vi "Register File.vi"(8 "Error In":errorcluster, 10 "Sequence File In":refnum<k7>, 11 "Application Manager In":refnum<k7>) -> (0 "Error out":errorcluster, 1 "Events":refnum<k27>[](array[refnum]), 2 "Sequence File Out":refnum<k7>, 3 "Application Manager Out":refnum<k7>)   [LabVIEW 2021, in "Seq Edit Quick Drop.lvlib"]
uses:
  Seq Edit Quick Drop.lvlib
  Connection Type.ctl
  Event Data.ctl
  Event Handler - Sequence View - Key Down.vi
  Event Handler - Sequence List - Key Up.vi
  Event Handler - Variables View - Key Down.vi
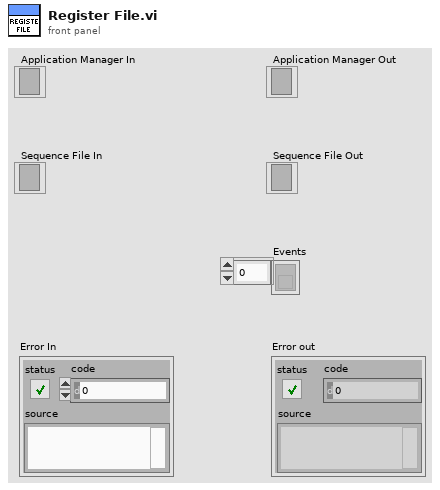
[diagram p1: front panel]
types:
  T1 = typedef "Seq Edit Quick Drop.lvlib/Event Data.ctl" = cluster{"Engine ID":string, "ID":i32}
  T2 = typedef "Seq Edit Quick Drop.lvlib/Connection Type.ctl" = enum16{"SequenceView", "SequenceList", "VariablesView"}
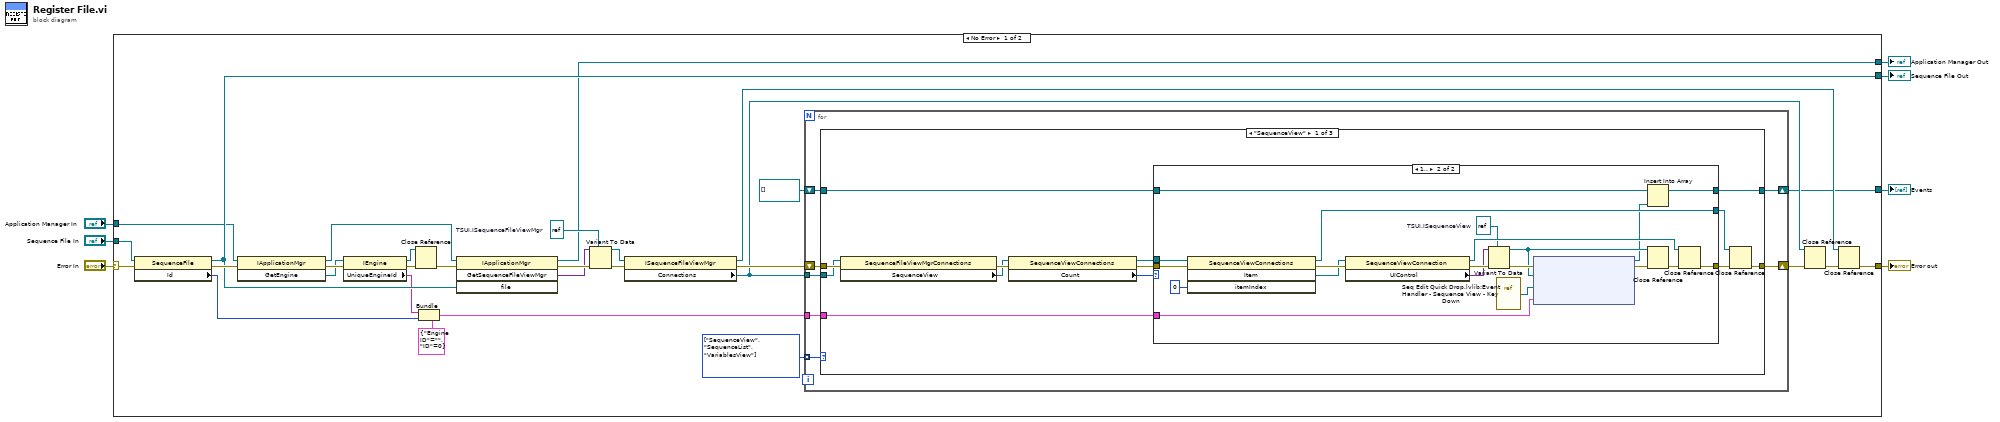
[diagram p0: block diagram]
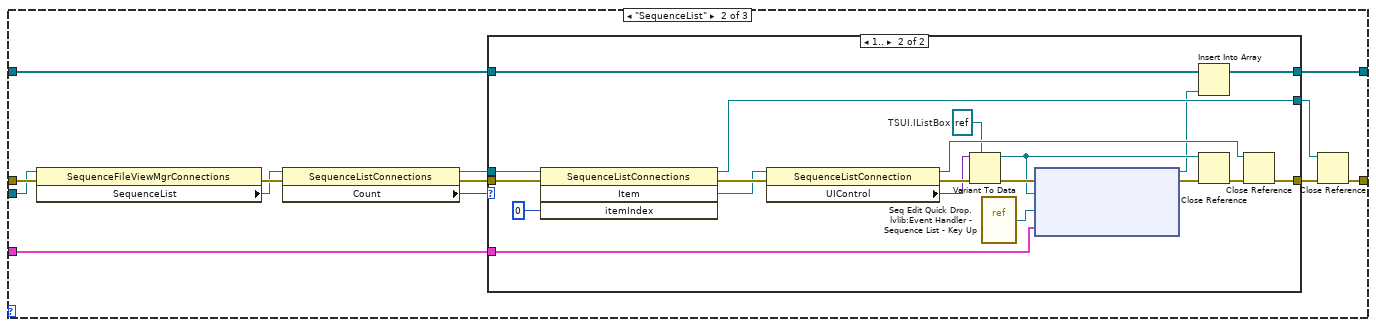
[diagram p3: hidden frame]
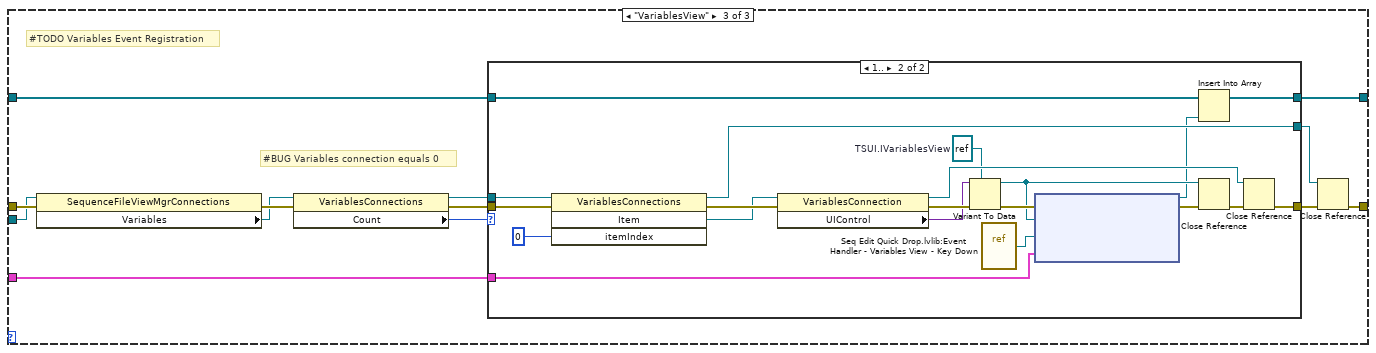
[diagram p5: hidden frame]
diagram:
  n1 = case shown="No Error" "Error In" {
    selector: "Error In" -> [w28 w155]
    tunnel: [w29 w155] -> w4
    tunnel: [w26 w154] -> w2
    tunnel: [w18 _] -> w3
    tunnel: "Application Manager In" -> [w17 w154]
    tunnel: "Sequence File In" -> [w20 w153]
    tunnel: [w35 w153] -> w1
    frame No Error {
      w25 = T2[] [enum."SequenceView", enum."SequenceList", enum."VariablesView"] items=["SequenceView", "SequenceList", "VariablesView"]
      w32 = refnum<k7> refnum  # TSUI.ISequenceFileViewMgr
      n2 = property class="SequenceFile"(reference=w20, error in=w28) -> (reference out=w35:refnum<k7>, error out=w36:errorcluster, "Id"=w10:i32)
      n3 = invoke class="IApplicationMgr" method="GetEngine"(reference=w17, error in=w36) -> (reference out=w15:refnum<k7>, error out=w37:errorcluster, "GetEngine"=w16:refnum<k7>)  [unwired: 1 in]
      n4 = property class="IEngine"(reference=w16, error in=w37) -> (reference out=w12:refnum<k7>, error out=w14:errorcluster, "UniqueEngineId"=w9:string)
      n5 = Close Reference(reference=w12, error in (no error)=w14) -> (error out=w13:errorcluster)
      n6 = Bundle(cluster=T1 {"Engine ID"="", "ID"=0}, "Engine ID"=w9, "ID"=w10) -> (w8:T1)
      n7 = invoke class="IApplicationMgr" method="GetSequenceFileViewMgr"(reference=w15, error in=w13, "file"=w35) -> (reference out=w26:refnum<k7>, error out=w34:errorcluster, "GetSequenceFileViewMgr"=w33:variant)  [unwired: 1 in, 1 out]
      n8 = Variant To Data(error in=w34, type=w32, Variant=w33) -> (data=w30:refnum<k7>, error out=w31:errorcluster)
      n9 = property class="ISequenceFileViewMgr"(reference=w30, error in=w31) -> (reference out=w27:refnum<k7>, error out=w24:errorcluster, "Connections"=w21:refnum<k7>)
      n10 = for {
        tunnel: w25 -> [w44] mode=indexing
        shift-right: [w41] -> w23
        shift-left: w24 -> [w42]
        tunnel: w21 -> [w43]
        shift-right: [w39] -> w18
        shift-left: refnum<k27>[] [] -> [w40]
        tunnel: w8 -> [w38]
        n11 = case shown="\"SequenceView\"" w44 {
          tunnel: w43 -> [w56 w92 w128]
          tunnel: w42 -> [w57 w93 w129]
          tunnel: [w47 w84 w120] -> w41
          tunnel: [w48 w82 w118] -> w39
          tunnel: w40 -> [w46 w83 w119]
          tunnel: w38 -> [w45 w81 w117]
          frame "SequenceView" {
            n12 = property class="SequenceFileViewMgrConnections"(reference=w56, error in=w57) -> (error out=w55:errorcluster, "SequenceView"=w54:refnum<k7>)  [unwired: 1 out]
            n13 = property class="SequenceViewConnections"(reference=w54, error in=w55) -> (reference out=w51:refnum<k7>, error out=w52:errorcluster, "Count"=w53:i32)
            n14 = case shown="1.." w53 {
              tunnel: w52 -> [w60 w77]
              tunnel: w51 -> [w59 w76]
              tunnel: [w60 w67] -> w50
              tunnel: [w59 w69] -> w49
              tunnel: [w58 w64] -> w48
              tunnel: w46 -> [w58 w65]
              tunnel: w45 -> [_ w61]
              frame Default {
              }
              frame 1.. {
                w73 = refnum<k7> refnum  # TSUI.ISequenceView
                n15 = invoke class="SequenceViewConnections" method="Item"(reference=w76, error in=w77, "itemIndex"=0) -> (reference out=w69:refnum<k7>, error out=w72:errorcluster, "Item"=w71:refnum<k7>)  [unwired: 1 in, 1 out]
                n16 = property class="SequenceViewConnection"(reference=w71, error in=w72) -> (reference out=w80:refnum<k7>, error out=w78:errorcluster, "UIControl"=w74:variant)
                n17 = Variant To Data(error in=w78, type=w73, Variant=w74) -> (data=w66:refnum<k7>, error out=w79:errorcluster)
                n18 = vi-ref "Seq Edit Quick Drop.lvlib:Event Handler - Sequence View - Key Down.vi"() -> ("vi reference"=w62:refnum<vi>)
                n19 = node(w79, w66, w62, w61) -> (w63:refnum<k27>, w70:errorcluster)  [unwired: 1 in]
                n20 = Insert Into Array(array=w65, new element=w63) -> (w64:refnum<k27>[])  [unwired: 1 in]
                n21 = Close Reference(reference=w66, error in (no error)=w70) -> (error out=w68:errorcluster)
                n22 = Close Reference(reference=w80, error in (no error)=w68) -> (error out=w67:errorcluster)
              }
            }
            n23 = Close Reference(reference=w49, error in (no error)=w50) -> (error out=w47:errorcluster)
          }
          frame "SequenceList" {
            n24 = property class="SequenceFileViewMgrConnections"(reference=w92, error in=w93) -> (error out=w91:errorcluster, "SequenceList"=w90:refnum<k7>)  [unwired: 1 out]
            n25 = property class="SequenceListConnections"(reference=w90, error in=w91) -> (reference out=w87:refnum<k7>, error out=w88:errorcluster, "Count"=w89:i32)
            n26 = case shown="1.." w89 {
              tunnel: w88 -> [w96 w113]
              tunnel: w87 -> [w95 w112]
              tunnel: [w96 w103] -> w86
              tunnel: [w95 w105] -> w85
              tunnel: w83 -> [w94 w101]
              tunnel: [w94 w99] -> w82
              tunnel: w81 -> [_ w98]
              frame Default {
              }
              frame 1.. {
                w109 = refnum<k7> refnum  # TSUI.IListBox
                n27 = invoke class="SequenceListConnections" method="Item"(reference=w112, error in=w113, "itemIndex"=0) -> (reference out=w105:refnum<k7>, error out=w108:errorcluster, "Item"=w107:refnum<k7>)  [unwired: 1 in, 1 out]
                n28 = property class="SequenceListConnection"(reference=w107, error in=w108) -> (reference out=w116:refnum<k7>, error out=w114:errorcluster, "UIControl"=w110:variant)
                n29 = Variant To Data(error in=w114, type=w109, Variant=w110) -> (data=w102:refnum<k7>, error out=w115:errorcluster)
                n30 = vi-ref "Seq Edit Quick Drop.lvlib:Event Handler - Sequence List - Key Up.vi"() -> ("vi reference"=w97:refnum<vi>)
                n31 = node(w115, w102, w97, w98) -> (w100:refnum<k27>, w106:errorcluster)  [unwired: 1 in]
                n32 = Insert Into Array(array=w101, new element=w100) -> (w99:refnum<k27>[])  [unwired: 1 in]
                n33 = Close Reference(reference=w102, error in (no error)=w106) -> (error out=w104:errorcluster)
                n34 = Close Reference(reference=w116, error in (no error)=w104) -> (error out=w103:errorcluster)
              }
            }
            n35 = Close Reference(reference=w85, error in (no error)=w86) -> (error out=w84:errorcluster)
          }
          frame "VariablesView" {
            # "#BUG Variables connection equals 0"
            # "#TODO Variables Event Registration"
            n36 = property class="SequenceFileViewMgrConnections"(reference=w128, error in=w129) -> (error out=w127:errorcluster, "Variables"=w126:refnum<k7>)  [unwired: 1 out]
            n37 = property class="VariablesConnections"(reference=w126, error in=w127) -> (reference out=w123:refnum<k7>, error out=w124:errorcluster, "Count"=w125:i32)
            n38 = case shown="1.." w125 {
              tunnel: w124 -> [w132 w149]
              tunnel: w123 -> [w131 w148]
              tunnel: [w132 w139] -> w122
              tunnel: [w131 w141] -> w121
              tunnel: w119 -> [w130 w137]
              tunnel: [w130 w135] -> w118
              tunnel: w117 -> [_ w134]
              frame Default {
              }
              frame 1.. {
                w145 = refnum<k7> refnum  # TSUI.IVariablesView
                n39 = invoke class="VariablesConnections" method="Item"(reference=w148, error in=w149, "itemIndex"=0) -> (reference out=w141:refnum<k7>, error out=w144:errorcluster, "Item"=w143:refnum<k7>)  [unwired: 1 in, 1 out]
                n40 = property class="VariablesConnection"(reference=w143, error in=w144) -> (reference out=w152:refnum<k7>, error out=w150:errorcluster, "UIControl"=w146:variant)
                n41 = Variant To Data(error in=w150, type=w145, Variant=w146) -> (data=w138:refnum<k7>, error out=w151:errorcluster)
                n42 = vi-ref "Seq Edit Quick Drop.lvlib:Event Handler - Variables View - Key Down.vi"() -> ("vi reference"=w133:refnum<vi>)
                n43 = node(w151, w138, w133, w134) -> (w136:refnum<k27>, w142:errorcluster)  [unwired: 1 in]
                n44 = Insert Into Array(array=w137, new element=w136) -> (w135:refnum<k27>[])  [unwired: 1 in]
                n45 = Close Reference(reference=w138, error in (no error)=w142) -> (error out=w140:errorcluster)
                n46 = Close Reference(reference=w152, error in (no error)=w140) -> (error out=w139:errorcluster)
              }
            }
            n47 = Close Reference(reference=w121, error in (no error)=w122) -> (error out=w120:errorcluster)
          }
        }
      }
      n48 = Close Reference(reference=w21, error in (no error)=w23) -> (error out=w22:errorcluster)
      n49 = Close Reference(reference=w27, error in (no error)=w22) -> (error out=w29:errorcluster)
    }
    frame Error {
    }
  }
  "Error out" <- w4
  "Events" <- w3
  "Application Manager Out" <- w2
  "Sequence File Out" <- w1
